vi "Read Single Measurement (Power).vi"(0 "VISA resource name":refnum<visa-resource-name>, 5 "Maximum Time (10000 ms)":i32=10000, 11 "error in (no error)":errorcluster) -> (2 "Power Factor":dbl, 3 "Reactive AC Power":dbl, 4 "VISA resource name out":refnum<visa-resource-name>, 6 "DC Power":dbl, 8 "Real AC Power":dbl, 10 "Apparent AC Power":dbl, 14 "Total Power":dbl, 15 "error out":errorcluster)   [LabVIEW 2020, in "Agilent 681x Series.lvlib"]
doc: "Initiates and reads a power measurement.\n\n<B>Note:</B>\n\nThis VI changes the <B>Trigger Source</B> to <B>Bus</B> and uses a software trigger after the instrument is initiated. If you want to control the triggering and other features, please use the low level VIs."
uses:
  <instrlib>/Agilent 681x Series/Agilent 681x Series.lvlib
  <instrlib>/Agilent 681x Series/Public/Data/Low Level/Fetch Single Measurement (Power).vi
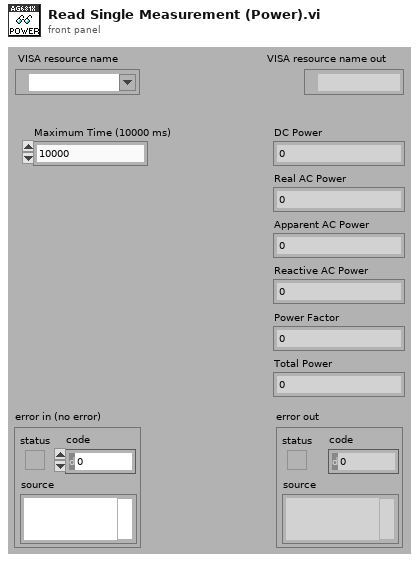
[diagram p1: front panel]
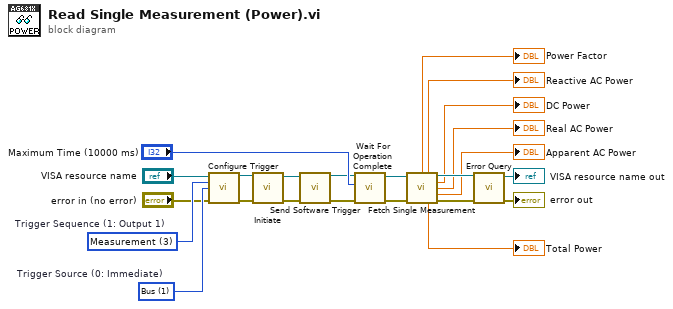
[diagram p0: block diagram]
diagram:
  w9 = 1 items=["Immediate", "Bus", "External", "Phase", "Trigger Out"]  # Trigger Source (0: Immediate)
  w10 = 3 items=["Output"=1, "Synchronous Source"=2, "Measurement"=3]  # Trigger Sequence (1: Output 1)
  n1 = call <instrlib>:"Configure Trigger.vi"("VISA resource name"="VISA resource name", "Trigger Sequence (1: Output 1)"=w10, "Trigger Source (0: Immediate)"=w9, "error in (no error)"="error in (no error)") -> ("VISA resource name out"=w7:refnum<visa-resource-name>, "error out"=w8:errorcluster)  [unwired: 10 in]
  n2 = call <instrlib>:"Initiate.vi"("error in (no error)"=w8, "VISA resource name"=w7) -> ("error out"=w6:errorcluster, "VISA resource name out"=w5:refnum<visa-resource-name>)  [unwired: 8 in]
  n3 = call <instrlib>:"Send Software Trigger.vi"("VISA resource name"=w5, "error in (no error)"=w6) -> ("VISA resource name out"=w4:refnum<visa-resource-name>, "error out"=w3:errorcluster)  [unwired: 12 in]
  n4 = call <instrlib>:"Wait For Operation Complete.vi"("error in (no error)"=w3, "Maximum Time (10000 ms)"="Maximum Time (10000 ms)", "VISA resource name"=w4) -> ("error out"=w21:errorcluster, "VISA resource name out"=w22:refnum<visa-resource-name>)  [unwired: 7 in]
  n5 = call-poly <instrlib>:"Fetch Single Measurement.vi"("VISA resource name"=w22, "error in (no error)"=w21) -> ("Power Factor"=→"Power Factor":dbl, "Reactive Power"=→"Reactive AC Power":dbl, "VISA resource name out"=w20:refnum<visa-resource-name>, "DC Power"=→"DC Power":dbl, "Real Power"=→"Real AC Power":dbl, "Apparent Power"=→"Apparent AC Power":dbl, "Total Power"=→"Total Power":dbl, "error out"=w19:errorcluster)  [unwired: 6 in]
  n6 = call <instrlib>:"Error Query.vi"("error in (no error)"=w19, "VISA resource name"=w20) -> ("error out"=→"error out":errorcluster, "VISA resource name out"=→"VISA resource name out":refnum<visa-resource-name>)  [unwired: 6 in, 2 out]
